vi "Message type to WAMP code value.vi"(3 "Message Type":T1) -> (1 "WAMP Numeric value":u8)   [LabVIEW 2020, in "wamplv.lvlib"]
uses:
  wamplv.lvlib
  TypeDefs/WAMP Message Codes.ctl
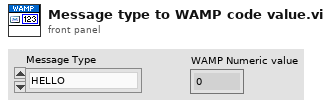
[diagram p1: front panel]
types:
  T1 = typedef "wamplv.lvlib/WAMP Message Codes.ctl" = enum8{"HELLO", "WELCOME", "CHALLENGE", "AUTHENTICATE", "ABORT", "GOODBYE", "ERROR", "PUBLISH", "PUBLISHED", "SUBSCRIBE", "SUBSCRIBED", "UNSUBSCRIBE", "UNSUBSCRIBED", "EVENT", "CALL", "RESULT", "REGISTER", "REGISTERED", "UNREGISTER", "UNREGISTERED", "INVOCATION", "YIELD"}
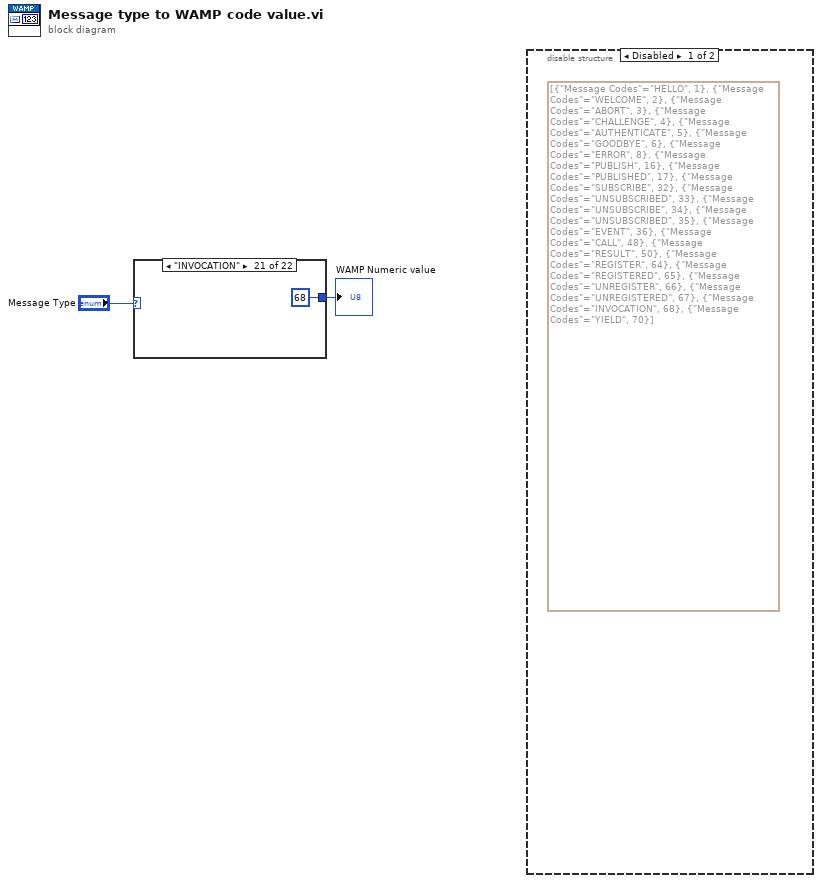
[diagram p0: block diagram]
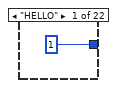
[diagram p3: hidden frame]
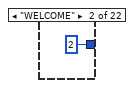
[diagram p4: hidden frame]
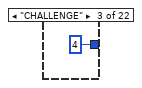
[diagram p5: hidden frame]
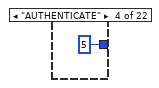
[diagram p6: hidden frame]
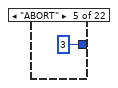
[diagram p7: hidden frame]
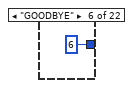
[diagram p8: hidden frame]
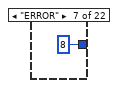
[diagram p9: hidden frame]
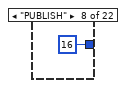
[diagram p10: hidden frame]
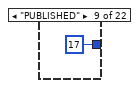
[diagram p11: hidden frame]
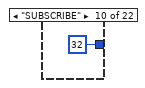
[diagram p12: hidden frame]
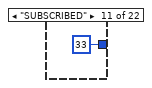
[diagram p13: hidden frame]
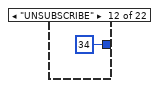
[diagram p14: hidden frame]
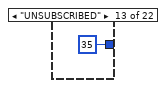
[diagram p15: hidden frame]
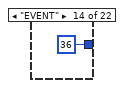
[diagram p16: hidden frame]
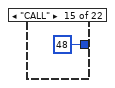
[diagram p17: hidden frame]
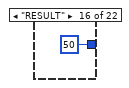
[diagram p18: hidden frame]
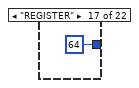
[diagram p19: hidden frame]
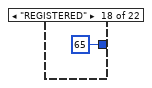
[diagram p20: hidden frame]
diagram:
  n1 = case shown="\"INVOCATION\"" "Message Type" {
    tunnel: [u8 1 u8 2 u8 4 u8 5 u8 3 u8 6 u8 8 u8 16 u8 17 u8 32 u8 33 u8 34 u8 35 u8 36 u8 48 u8 50 u8 64 u8 65 u8 66 u8 67 u8 68 u8 70] -> w1
    frame "HELLO" {
    }
    frame "WELCOME" {
    }
    frame "CHALLENGE" {
    }
    frame "AUTHENTICATE" {
    }
    frame "ABORT" {
    }
    frame "GOODBYE" {
    }
    frame "ERROR" {
    }
    frame "PUBLISH" {
    }
    frame "PUBLISHED" {
    }
    frame "SUBSCRIBE" {
    }
    frame "SUBSCRIBED" {
    }
    frame "UNSUBSCRIBE" {
    }
    frame "UNSUBSCRIBED" {
    }
    frame "EVENT" {
    }
    frame "CALL" {
    }
    frame "RESULT" {
    }
    frame "REGISTER" {
    }
    frame "REGISTERED" {
    }
    frame "UNREGISTER" {
    }
    frame "UNREGISTERED" {
    }
    frame "INVOCATION" {
    }
    frame "YIELD" {
    }
  }
  "WAMP Numeric value" <- w1
  n2 = disable-structure shown="Disabled" {
    frame Disabled {
      (unwired) cluster{"Message Codes":T1, u8}[] [{"Message Codes"=enum."HELLO", 1}, {"Message Codes"=enum."WELCOME", 2}, {"Message Codes"=enum."ABORT", 3}, {"Message Codes"=enum."CHALLENGE", 4}, {"Message Codes"=enum."AUTHENTICATE", 5}, {"Message Codes"=enum."GOODBYE", 6}, {"Message Codes"=enum."ERROR", 8}, {"Message Codes"=enum."PUBLISH", 16}, {"Message Codes"=enum."PUBLISHED", 17}, {"Message Codes"=enum."SUBSCRIBE", 32}, {"Message Codes"=enum."UNSUBSCRIBED", 33}, {"Message Codes"=enum."UNSUBSCRIBE", 34}, {"Message Codes"=enum."UNSUBSCRIBED", 35}, {"Message Codes"=enum."EVENT", 36}, {"Message Codes"=enum."CALL", 48}, {"Message Codes"=enum."RESULT", 50}, {"Message Codes"=enum."REGISTER", 64}, {"Message Codes"=enum."REGISTERED", 65}, {"Message Codes"=enum."UNREGISTER", 66}, {"Message Codes"=enum."UNREGISTERED", 67}, {"Message Codes"=enum."INVOCATION", 68}, {"Message Codes"=enum."YIELD", 70}] ("output cluster")
    }
    frame Enabled {
    }
  }
